vi "EEG_2021_099 2D arrays.vi"() -> ()   [LabVIEW 2022 SP3]
panel:
  out "appended array":dbl[](array[numeric])
  out "subarray":dbl[](array[numeric])
  out "size(s) 2":i32[](array[numeric])
  out "size(s)":i32
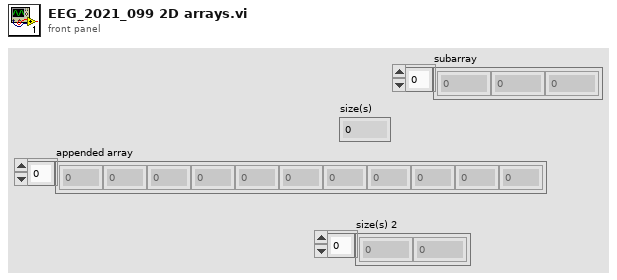
[diagram p1: front panel]
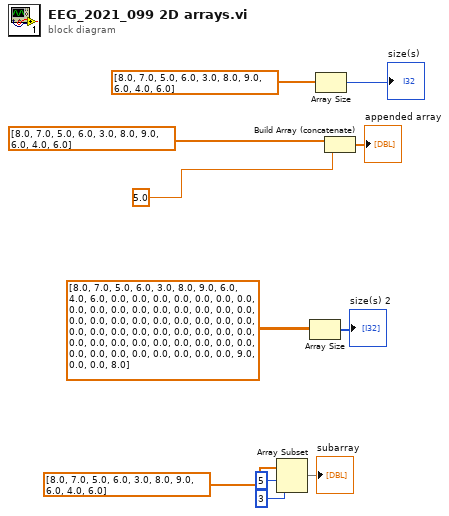
[diagram p0: block diagram]
diagram:
  n1 = Array Subset(array=dbl[] [8.0, 7.0, 5.0, 6.0, 3.0, 8.0, 9.0, 6.0, 4.0, 6.0], index=5, length=3) -> (→"subarray":dbl[])
  n2 = Array Size(array=dbl[][] [[8.0, 7.0, 5.0, 6.0, 3.0, 8.0, 9.0, 6.0, 4.0, 6.0, 0.0, 0.0, 0.0], [0.0, 0.0, 0.0, 0.0, 0.0, 0.0, 0.0, 0.0, 0.0, 0.0, 0.0, 0.0, 0.0], [0.0, 0.0, 0.0, 0.0, 0.0, 0.0, 0.0, 0.0, 0.0, 0.0, 0.0, 0.0, 0.0], [0.0, 0.0, 0.0, 0.0, 0.0, 0.0, 0.0, 0.0, 0.0, 0.0, 0.0, 0.0, 0.0], [0.0, 0.0, 0.0, 0.0, 0.0, 0.0, 0.0, 0.0, 0.0, 9.0, 0.0, 0.0, 8.0]]) -> (size(s)=→"size(s) 2":i32[])
  n3 = Array Size(array=dbl[] [8.0, 7.0, 5.0, 6.0, 3.0, 8.0, 9.0, 6.0, 4.0, 6.0]) -> (size(s)=→"size(s)":i32)
  n4 = Build Array (concatenate)(dbl[] [8.0, 7.0, 5.0, 6.0, 3.0, 8.0, 9.0, 6.0, 4.0, 6.0], 5.0) -> (→"appended array":dbl[])
